vi "Histogram2DManual2001.vi"   [LabVIEW 2013]
uses:
  <vilib>/Heliosphere Research LLC/Advanced Plotting Toolkit/api_plotting/Histogram2D_Manual.vi
  <vilib>/Heliosphere Research LLC/Advanced Plotting Toolkit/Advanced Plotting Toolkit.lvlib
types:
  T1 = typedef "Advanced Plotting Toolkit.lvlib/PlotID.ctl" = i32
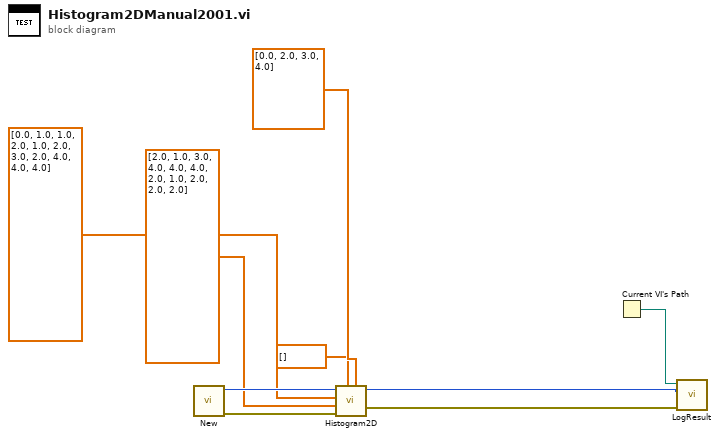
[diagram p0: block diagram]
diagram:
  n1 = call <vilib>:"New.vi"() -> ("error out"=w7:errorcluster, "Plot ID"=w8:T1)  [unwired: 10 in]
  n2 = call-poly <vilib>:"Histogram2D.vi"("Y Bin Edges"=dbl[] [0.0, 2.0, 3.0, 4.0] ("X Bin Edges"), "X Bin Edges"=dbl[] [], "error in (no error)"=w7, "Y Data"=dbl[] [2.0, 1.0, 3.0, 4.0, 4.0, 4.0, 2.0, 1.0, 2.0, 2.0, 2.0] ("X Data"), "X Data"=dbl[] [0.0, 1.0, 1.0, 2.0, 1.0, 2.0, 3.0, 2.0, 4.0, 4.0, 4.0], "Plot ID"=w8) -> ("error out"=w5:errorcluster, "Plot ID Out"=w6:T1)  [unwired: 4 in]
  n3 = Current VI's Path() -> (path=w9:path)
  n4 = call "LogResult.vi"("Test Result"=w5, "Test Artifact"=w6, "VI Path"=w9) -> ()  [unwired: 9 in]
